vi "Double Decoder.vi"(8 "error in (no error)":errorcluster, 9 "Array":u8[](array[numeric]) format="%02x", 10 "Key":i32=-1) -> (0 "error out":errorcluster, 1 "array w/ subset deleted":u8[](array[numeric]), 2 "Read Key":i32, 3 "Double":dbl)   [LabVIEW 2018]
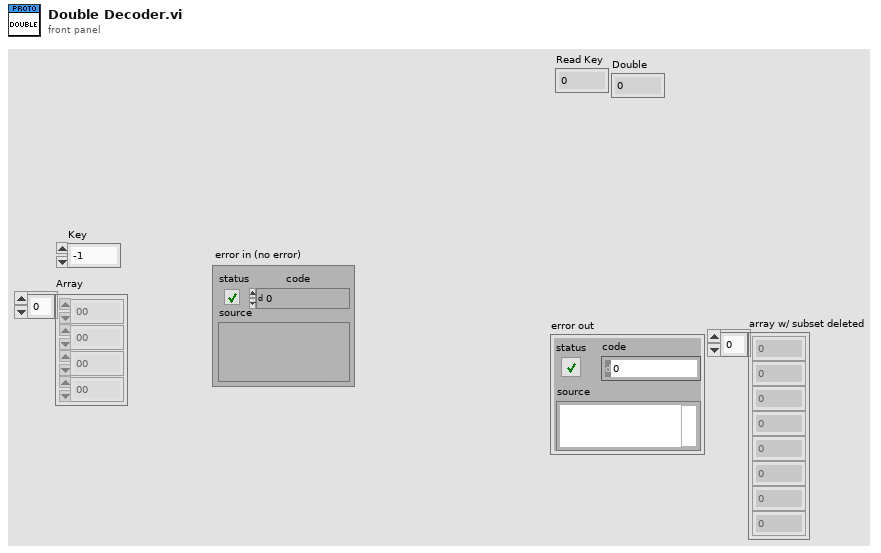
[diagram p1: front panel]
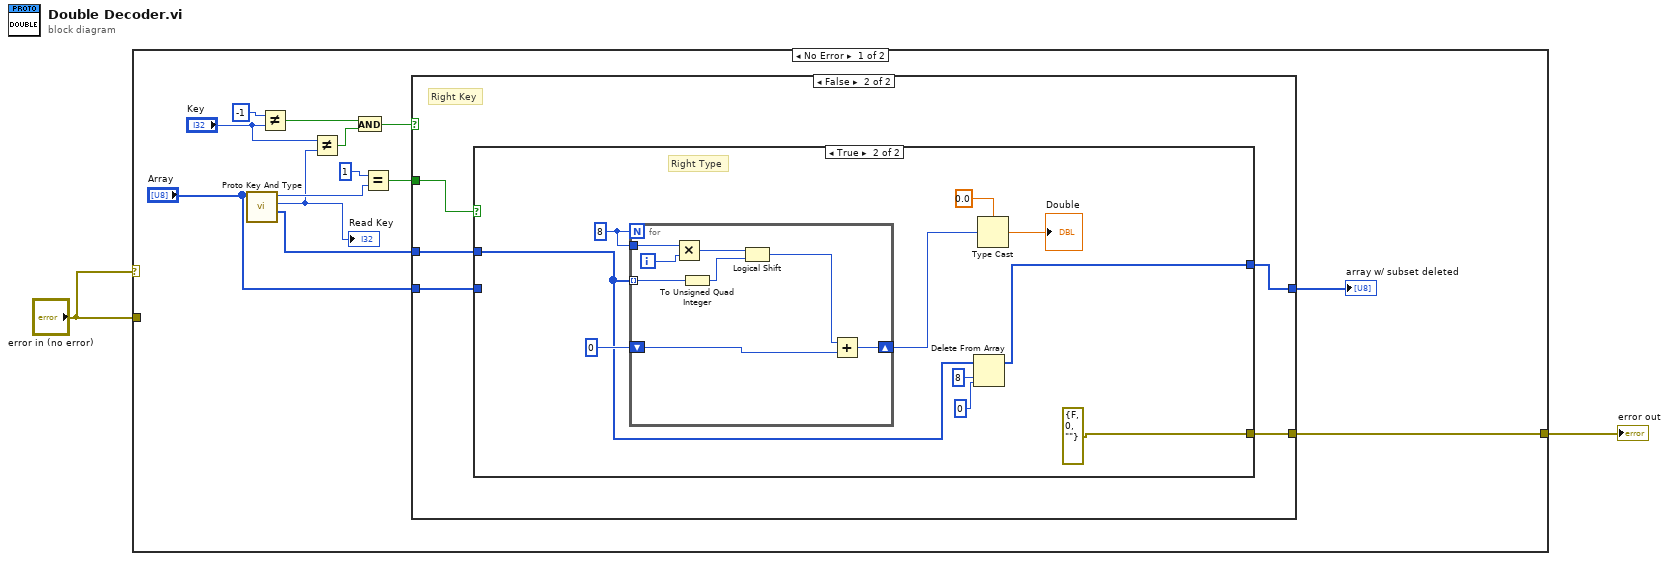
[diagram p0: block diagram]
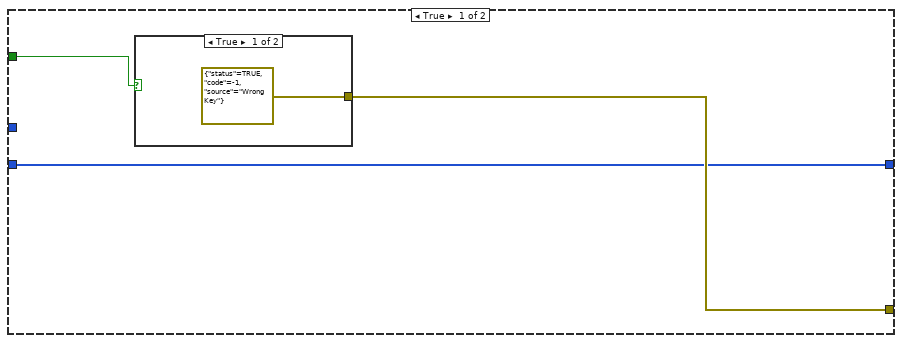
[diagram p2: hidden frame]
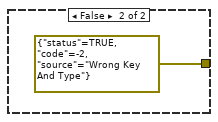
[diagram p3: hidden frame]
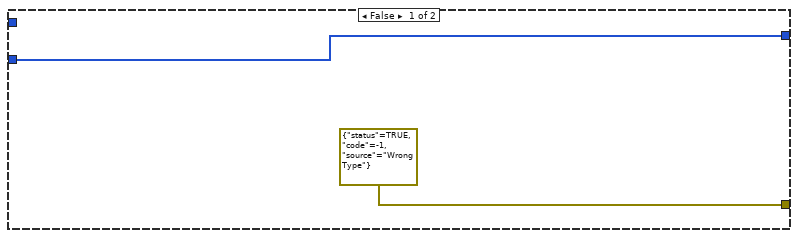
[diagram p4: hidden frame]
diagram:
  n1 = case shown="No Error" "error in (no error)" {
    tunnel: "error in (no error)" -> [_ w46]
    tunnel: [w3 w46] -> w1
    frame No Error {
      n2 = call "Proto Key And Type.vi"("Array"="Array") -> ("array w/ subset deleted"=w15:u8[], "Key"=w4:i32, "Type"=w7:i32)  [unwired: 8 in]
      "Read Key" <- w4
      n3 = Not Equal?(x=-1, y="Key") -> (x != y?=w12:bool)
      n4 = Not Equal?(x="Key", y=w4) -> (x != y?=w10:bool)
      n5 = And(x=w12, y=w10) -> (x .and. y?=w9:bool)
      n6 = Equal?(x=1, y=w7) -> (x = y?=w6:bool)
      n7 = case shown="False" w9 {
        tunnel: w15 -> [_ w25]
        tunnel: "Array" -> [w16 w24]
        tunnel: w6 -> [w18 w23]
        tunnel: [w17 w22] -> w3
        tunnel: [w16 w21] -> w5
        frame True {
          n8 = case shown="True" w18 {
            tunnel: [errorcluster {"status"=TRUE, "code"=-1, "source"="Wrong Key"} ("error in (no error)") errorcluster {"status"=TRUE, "code"=-2, "source"="Wrong Key And Type"} ("error in (no error)")] -> w17
            frame True {
            }
            frame False {
            }
          }
        }
        frame False {
          # "Right Key"
          n9 = case shown="True" w23 {
            tunnel: [errorcluster {"status"=TRUE, "code"=-1, "source"="Wrong Type"} ("error in (no error)") errorcluster {"status"=FALSE, "code"=0, "source"=""} ("error in (no error)")] -> w22
            tunnel: w25 -> [_ w34]
            tunnel: [w26 w33] -> w21
            tunnel: w24 -> [w26 _]
            frame False {
            }
            frame True {
              w32 = 8
              # "Right Type"
              n10 = for {
                N: w32 -> [_]
                tunnel: w34 -> [w39] mode=indexing
                shift-right: [w45] -> w30
                shift-left: u64 0 -> [w40]
                tunnel: w32 -> [w43]
                i -> [w44]
                n11 = Multiply(x=w43, y=w44) -> (x*y=w42:i32)
                n12 = To Unsigned Quad Integer(1:w39) -> (0:w38:u64)
                n13 = Logical Shift(y=w42, x=w38) -> (x << y=w41:u64)
                n14 = Add(x=w41, y=w40) -> (x+y=w45:u64)
              }
              n15 = Delete From Array(array=w34, length=8, index=0) -> (array with subset deleted=w33:u8[])  [unwired: 1 out]
              n16 = Type Cast(type=0.0, x=w30) -> (*(type *) &x=→"Double":dbl)
            }
          }
        }
      }
      "array w/ subset deleted" <- w5
    }
    frame Error {
    }
  }
  "error out" <- w1
